vi "GlobalInit.vi"(1 "错误输入（无错误）":errorcluster) -> (0 "错误输出":errorcluster)   [LabVIEW 2018]
uses:
  InOut/Reslut.vi
  AllPath.vi
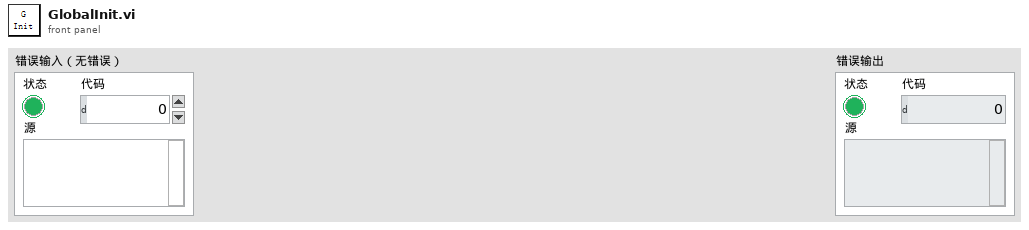
[diagram p1: front panel]
types:
  T1 = cluster{"任务":cluster{"功率任务":bool, "能量任务":bool, "时间波形任务":bool, "光谱任务":bool, "偏振任务":bool, "近远场任务":bool}, "通信":cluster{"功率通信":bool, "能量通信":bool, "时间波形通信":bool, "光谱通信":bool, "偏振通信":bool, "近远场通信":bool}}
  T2 = cluster{"能量计结果":string, "功率计结果":string, "能量计单位":string, " 功率计单位":string}
  T3 = cluster{" 偏振方向":string, "偏振度":string, " 偏振方向 单位 ":string, "偏振度单位":string}
  T4 = cluster{"能量/功率":path, " 示波器":path, " 光谱仪":path, "偏振":path, "近远场":cluster{" 近场图片":path, " 远场图片":path, "发散角数据":path}, "参数":path, " 基路径":path, "文件名信息":path}
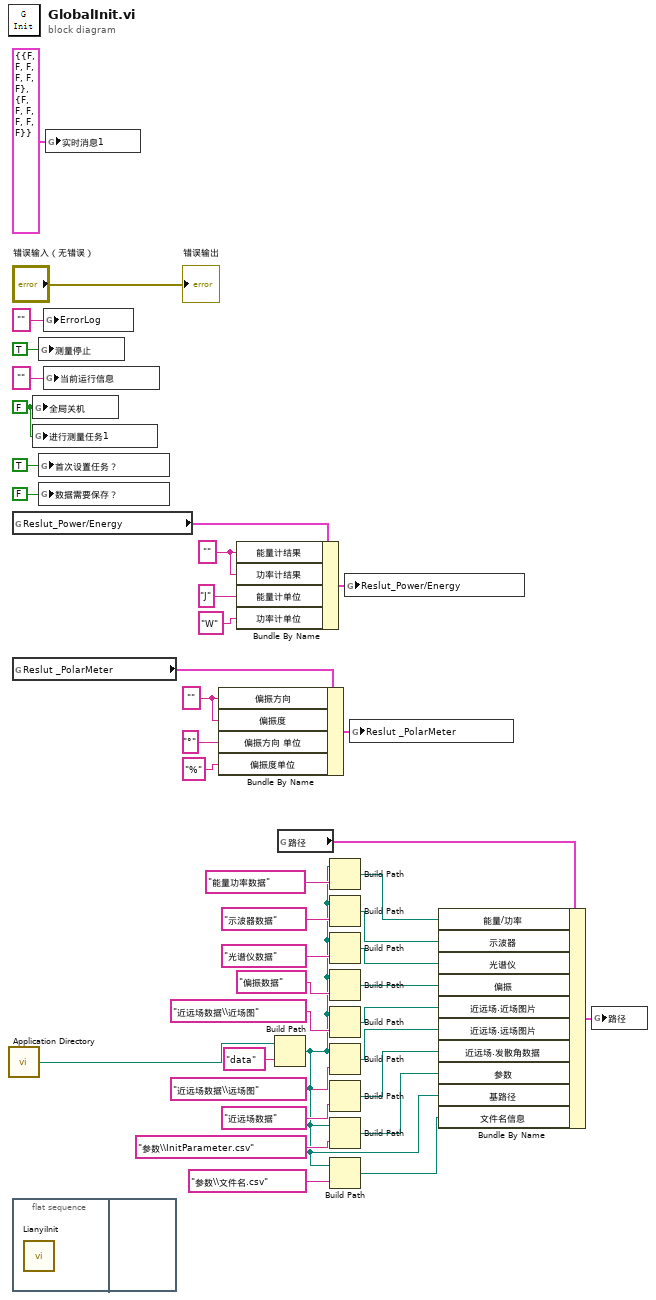
[diagram p0: block diagram]
diagram:
  w2 = ""
  w6 = ""
  w7 = FALSE ("全局关机")
  n1 = call <vilib>:"Application Directory.vi"() -> ("Application Directory"=w31:path)
  n2 = global read "Reslut.vi" "Reslut_Power/Energy"() -> (w36:T2)
  n3 = global read "Reslut.vi" "Reslut _PolarMeter"() -> (w5:T3)
  n4 = flat-sequence {
    frame #0 {
      n5 = call "LianyiInit.vi"() -> ()  [unwired: 12 in]
    }
    frame #1 {
    }
  }
  n6 = global write "参数.vi" "全局关机"(w7) -> ()
  n7 = global write "参数.vi" "进行测量任务1"(w7) -> ()
  n8 = global write "参数.vi" "测量停止"(TRUE ("测量停止")) -> ()
  n9 = global write "globalMessage.vi" "首次设置任务？"(TRUE ("首次设置任务？")) -> ()
  n10 = global write "globalMessage.vi" "数据需要保存？"(FALSE ("数据是否保存？")) -> ()
  n11 = global write "参数.vi" "ErrorLog"("" ("ErrorLog")) -> ()
  n12 = global write "globalMessage.vi" "当前运行信息"("" ("当前运行信息")) -> ()
  n13 = global write "globalMessage.vi" "实时消息1"(T1 {"任务"={"功率任务"=FALSE, "能量任务"=FALSE, "时间波形任务"=FALSE, "光谱任务"=FALSE, "偏振任务"=FALSE, "近远场任务"=FALSE}, "通信"={"功率通信"=FALSE, "能量通信"=FALSE, "时间波形通信"=FALSE, "光谱通信"=FALSE, "偏振通信"=FALSE, "近远场通信"=FALSE}} ("实时消息")) -> ()
  n14 = Bundle By Name(cluster=w5, "偏振方向"=w2, "偏振度"=w2, "偏振方向 单位"="°", "偏振度单位"="%") -> (w1:T3)
  n15 = Bundle By Name(cluster=w36, "能量计结果"=w6, "功率计结果"=w6, "能量计单位"="J", "功率计单位"="W") -> (w35:T2)
  n16 = Build Path(base path=w31, name or relative path="data" ("名称或相对路径")) -> (appended path=w11:path)
  n17 = global read "AllPath.vi" "路径"() -> (w32:T4)
  n18 = Build Path(base path=w11, name or relative path="能量功率数据" ("名称或相对路径")) -> (appended path=w29:path)
  n19 = Build Path(base path=w11, name or relative path="示波器数据" ("名称或相对路径")) -> (appended path=w26:path)
  n20 = Build Path(base path=w11, name or relative path="光谱仪数据" ("名称或相对路径")) -> (appended path=w24:path)
  n21 = Build Path(base path=w11, name or relative path="偏振数据" ("名称或相对路径")) -> (appended path=w22:path)
  n22 = Build Path(base path=w11, name or relative path="近远场数据\\近场图" ("名称或相对路径")) -> (appended path=w20:path)
  n23 = Build Path(base path=w11, name or relative path="近远场数据\\远场图" ("名称或相对路径")) -> (appended path=w18:path)
  n24 = Build Path(base path=w11, name or relative path="近远场数据" ("名称或相对路径")) -> (appended path=w16:path)
  n25 = Build Path(base path=w11, name or relative path="参数\\InitParameter.csv" ("名称或相对路径")) -> (appended path=w15:path)
  n26 = Build Path(base path=w11, name or relative path="参数\\文件名.csv" ("名称或相对路径")) -> (appended path=w12:path)
  n27 = global write "Reslut.vi" "Reslut_Power/Energy"(w35) -> ()
  n28 = global write "Reslut.vi" "Reslut _PolarMeter"(w1) -> ()
  n29 = Bundle By Name(cluster=w32, "能量/功率"=w29, "示波器"=w26, "光谱仪"=w24, "偏振"=w22, "近远场.近场图片"=w20, "近远场.远场图片"=w18, "近远场.发散角数据"=w16, "参数"=w15, "基路径"=w11, "文件名信息"=w12) -> (w13:T4)
  n30 = global write "AllPath.vi" "路径"(w13) -> ()
  "错误输出" <- "错误输入（无错误）"
